vi "Index.vi"(8 "error in (no error)":errorcluster, 10 "Index":i32, 11 "String Array in":refnum<class "String Array.lvclass">) -> (0 "error out":errorcluster, 3 "Indexed element":refnum<class "Generic Data.lvclass">)   [LabVIEW 2020, in "Data.lvlib" / "String Array.lvclass"]
doc: "Index an element from 'Generic Data in'.\nThis implementation returns a generic String class with the indexed string."
uses:
  String Array.lvclass
  Generic Data.lvclass
  String Array.lvclass/String Array.ctl
  String/String.lvclass/String.ctl
  String/String.lvclass
  C:/Users/Henri/OneDrive/LabVIEW/Framework/Data/Generic Data/Generic Data.lvclass
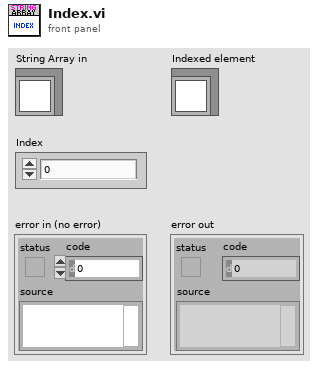
[diagram p1: front panel]
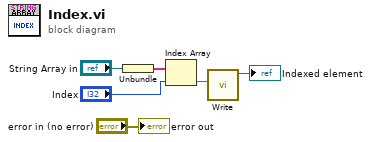
[diagram p0: block diagram]
diagram:
  n1 = Unbundle("String Array in") -> (w5:string[])
  n2 = Index Array(array=w5, index="Index") -> (element=w3:string)
  n3 = call "Write.vi"("String"=w3) -> ("String out"=→"Indexed element":refnum<class "String.lvclass">)  [unwired: 10 in]
  "error out" <- "error in (no error)"
